vi "Data Storage (16xI16).vi"(0 "data in":T2=[0, 0, 0, 0, 0, 0, 0, 0, 0, 0, 0, 0, 0, 0, 0, 0], 1 "input valid":bool, 3 "memory mode (F)":bool, 4 "priority (balanced)":T1, 5 "burst length (128)":u16=128, 6 "bypass DRAM FIFO (F)":bool, 8 "DRAM Memory":refnum<k21>, 9 "ready for output (T)":bool=TRUE, 10 "Memory Size":u32, 12 "DRAM Ready":bool, 13 "keep data (F)":bool, 14 "reset":bool, 15 "# of bits":u64) -> (18 "reset done":bool, 19 "ready for input":bool, 20 "data out":T2, 21 "output valid":bool)   [LabVIEW 2018, in "Streaming FPGA.lvlib"]
doc: "Data Storage using the data type provided by the <B>Data Type (16xI16).ctl</B>. This storage can act as a FIFO (<B>memory mode</B> is false) or as a Memory (<B>memory mode</B> is true).\n\nWhen the Data Storage is used in Memory mode, it must be written first by <B># of bits</B> booleans following a reset. No data output is returned during this write period. Once the Data Storage is written, the data output starts returning the <B># of bits</B> booleans stored in the memory, repeatedly. The <B>data in</B> input is an array of 16 I16s, representing 256 booleans, if <B># of bits</B> is not a multiple of 256 then padding booleans has to be used during the last input write operation, but these padding elements will be ignored. It is also possible to skip the Data Storage write period by setting the <B>keep data</B> input to true before applying the reset.\n\nThe Data Storage uses the memory resource provided on the <B>DRAM Memory</B> input for storing the data elements. The <B>DRAM Memory</B> memory resource must use DRAM implementation and the data type must be the type provided by the <B>Data Type (B256).ctl</B> (array of 256 booleans). The <B>Memory Size</B> must be the requested number of elements parameter of the memory resource. <B>DRAM Ready</B> must be set to true if the DRAM is ready. The <B>burst length</B> must be the DRAM read/write burst length the DRAM FIFO implementation should use (this must be less than the <B>Memory Size</B> and must be less than 508). Use the <B>priority</B> input to select which operations to favor in FIFO mode: the \"favor writes\" option gives priority to DRAM FIFO writes, the \"favor reads\" option gives priority to DRAM FIFO reads, the \"balanced\" option balances between DRAM FIFO reads and writes. Set the <B>bypass DRAM FIFO</B> input to true to disable the use of the DRAM in FIFO mode.\n\nIn FIFO mode the Data Storage can hold at least <B>Memory Size</B>+1024 data elements (16xI16s) in case the DRAM is enabled (<B>bypass DRAM FIFO</B> is false), and 1024 data elements (16xI16s) in case the DRAM is disabled (<B>bypass DRAM FIFO</B> is true)."
uses:
  Streaming FPGA.lvlib
  Data Type (16xI16).ctl
  Data Storage - DRAM FIFO Priority.ctl
  <instrlib>/_niInstr/Data Formatting/v1/FPGA/Private/Convert/U16 array to Boolean Array.vi
  <instrlib>/_niInstr/Data Formatting/v1/FPGA/Private/Convert/Boolean Array to U16 Array.vi
  <instrlib>/_niInstr/Data Formatting/v1/FPGA/niInstr Data Formatting v1 FPGA.lvlib
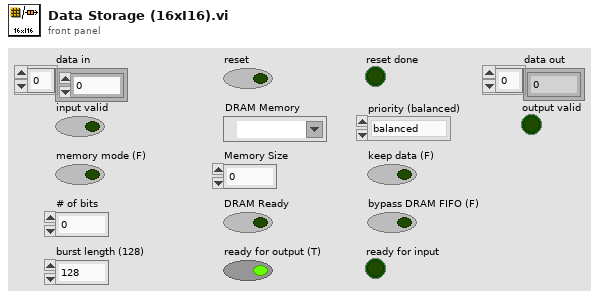
[diagram p1: front panel]
types:
  T1 = typedef "Streaming FPGA.lvlib/Data Storage - DRAM FIFO Priority.ctl" = enum16{"balanced", "favor writes", "favor reads"}
  T2 = typedef "Streaming FPGA.lvlib/Data Type (16xI16).ctl" = i16[]
  T3 = typedef "Streaming FPGA.lvlib/Data Type (B256).ctl" = bool[]
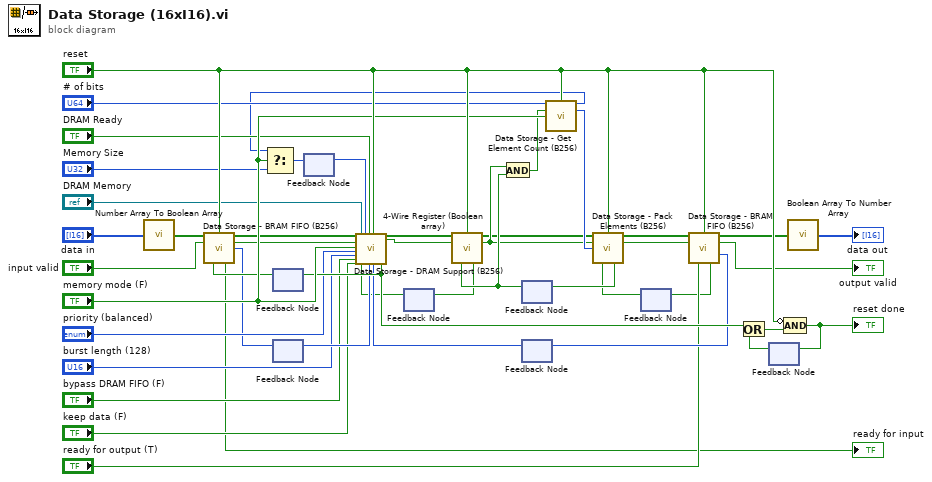
[diagram p0: block diagram]
diagram:
  n1 = call-poly <instrlib>:"Number Array To Boolean Array.vi"("data in"="data in") -> ("data out"=w15:bool[])  [unwired: 14 in]
  n2 = feedback #1() -> (w44:bool)  [unwired: 1 in]
  n3 = call "Data Storage - BRAM FIFO (B256).vi"("data in"=w15, "reset"="reset", "input valid"="input valid", "ready for output (T)"=w44) -> ("data out"=w11:T3, "output valid"=w10:bool, "# of elements to read"=w27:u32, "ready for input"=→"ready for input":bool)  [unwired: 7 in, 1 out]
  n4 = feedback-in #2(w27) -> ()
  n5 = feedback #2() -> (w42:u32)  [unwired: 1 in]
  n6 = feedback #3() -> (w23:u32)  [unwired: 1 in]
  n7 = feedback #4() -> (w6:bool)  [unwired: 1 in]
  n8 = feedback #5() -> (w8:bool)  [unwired: 1 in]
  n9 = feedback #6() -> (w28:u32)  [unwired: 1 in]
  n10 = call "Data Storage - DRAM Support (B256).vi"("data in"=w11, "input valid"=w10, "memory mode (F)"="memory mode (F)", "priority (balanced)"="priority (balanced)", "burst length (128)"="burst length (128)", "bypass DRAM FIFO (F)"="bypass DRAM FIFO (F)", "keep data (F)"="keep data (F)", "DRAM Memory"="DRAM Memory", "ready for output (T)"=w6, "Memory Size"=w23, "DRAM Ready"="DRAM Ready", "# of inputs available"=w42, "reset"="reset", "# of outputs ready for"=w28) -> ("ready for input"=w43:bool, "data out"=w1:T3, "output valid"=w4:bool)  [unwired: 11 in]
  n11 = feedback-in #1(w43) -> ()
  n12 = call "4-Wire Register (Boolean array).vi"("data in"=w1, "reset"="reset", "input valid"=w4, "ready for output (T)"=w8) -> ("data out"=w3:bool[], "output valid"=w5:bool, "ready for input"=w7:bool)  [unwired: 9 in]
  n13 = feedback-in #4(w7) -> ()
  n14 = And(x=w5, y=w8) -> (x .and. y?=w17:bool)
  n15 = call "Data Storage - Get Element Count (B256).vi"("# of bits"="# of bits", "reset"="reset", "read enable"=w17, "bit counter enable"="memory mode (F)") -> ("memory size"=w18:u32, "bit count"=w20:u16)  [unwired: 10 in]
  n16 = Select(t=w18, s="memory mode (F)", f="Memory Size") -> (s? t:f=w21:u32)
  n17 = feedback-in #3(w21) -> ()
  n18 = feedback #7() -> (w29:bool)  [unwired: 1 in]
  n19 = call "Data Storage - Pack Elements (B256).vi"("data in"=w3, "reset"="reset", "input valid"=w5, "bit count"=w20, "ready for output (T)"=w29) -> ("data out"=w2:bool[], "output valid"=w9:bool, "ready for input"=w32:bool)  [unwired: 8 in]
  n20 = feedback-in #5(w32) -> ()
  n21 = call "Data Storage - BRAM FIFO (B256).vi"("data in"=w2, "reset"="reset", "input valid"=w9, "ready for output (T)"="ready for output (T)") -> ("data out"=w13:T3, "output valid"=→"output valid":bool, "# of elements to write"=w38:u32, "ready for input"=w31:bool)  [unwired: 7 in, 1 out]
  n22 = feedback-in #6(w38) -> ()
  n23 = feedback-in #7(w31) -> ()
  n24 = feedback #8() -> (w40:bool)  [unwired: 1 in]
  n25 = Or(x=w43, y=w40) -> (x .or. y?=w41:bool)
  n26 = Compound Arithmetic op=AND(invert "reset", w41) -> (w39:bool)
  "reset done" <- w39
  n27 = feedback-in #8(w39) -> ()
  n28 = call-poly <instrlib>:"Boolean Array To Number Array.vi"("data in"=w13) -> ("data out"=→"data out":u16[])  [unwired: 14 in]
